vi "Basic_main_1.vi"() -> ()   [LabVIEW 2026]
panel:
  out "output":dbl
  in  "constant":dbl
  in  "Input_range":dbl
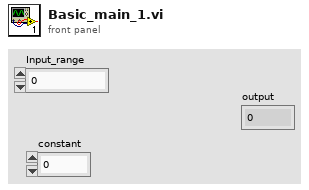
[diagram p1: front panel]
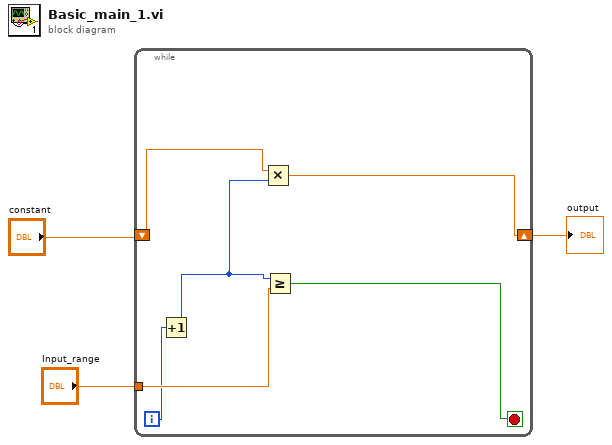
[diagram p0: block diagram]
diagram:
  n1 = while {
    tunnel: "Input_range" -> [w9]
    shift-right: [w6] -> w1
    shift-left: "constant" -> [w7]
    i -> [w4]
    stop <- w8 stop-if-true
    n2 = Increment(x=w4) -> (x+1=w5:i32)
    n3 = Multiply(x=w7, y=w5) -> (x*y=w6:dbl)
    n4 = Greater Or Equal?(x=w5, y=w9) -> (x >= y?=w8:bool)
  }
  "output" <- w1
